vi "Read LastIdentityQuery.vi"(8 "error in (no error)":errorcluster, 11 "SqlMapper in":refnum<class "SqlMapper.lvclass">) -> (0 "error out":errorcluster, 2 "LastIdentityQuery":string="select @@IDENTITY id", 3 "SqlMapper out":refnum<class "SqlMapper.lvclass">)   [LabVIEW 2020, in "ORM.lvlib" / "SqlMapper.lvclass"]
uses:
  SqlMapper.lvclass
  DbConnection/DbConnection.lvclass
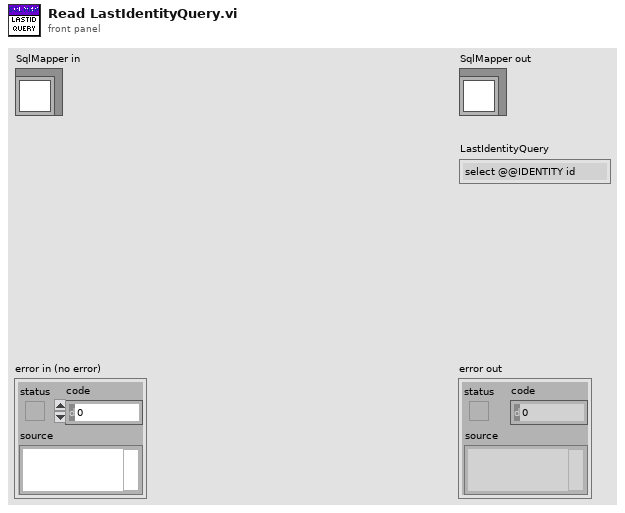
[diagram p1: front panel]
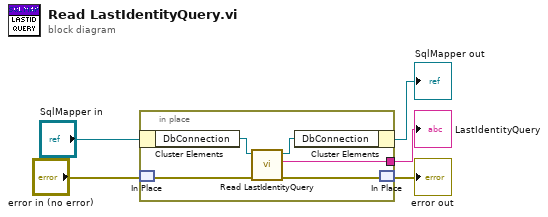
[diagram p0: block diagram]
diagram:
  n1 = in-place {
    in-place-border: [w10] -> w1
    n2 = in-place-cluster #1("SqlMapper in") -> ("DbConnection"=w9:refnum<class "DbConnection.lvclass">)
    n3 = in-place-match #2("error in (no error)") -> (w8:errorcluster)
    n4 = call "Read LastIdentityQuery.vi"("error in (no error)"=w8, "DbConnection in"=w9) -> ("error out"=w7:errorcluster, "LastIdentityQuery"=w10:string, "DbConnection out"=w6:refnum<class "DbConnection.lvclass">)  [unwired: 7 in]
    n5 = in-place-cluster #1("DbConnection"=w6) -> (→"SqlMapper out":refnum<class "SqlMapper.lvclass">)
    n6 = in-place-match #2(w7) -> (→"error out":errorcluster)
  }
  "LastIdentityQuery" <- w1
